vi "Credit Update.vi"(8 "error in (no error)":errorcluster, 10 "Credit":dbl, 11 "UI Actor in":refnum<class "UI Actor.lvclass">) -> (0 "error out":errorcluster, 3 "UI Actor out":refnum<class "UI Actor.lvclass">)   [LabVIEW 2020, in "UI Actor.lvlib" / "UI Actor.lvclass"]
uses:
  UI Actor.lvclass
  UI Actor.lvclass/UI Actor.ctl
  Msg Messages/Update MSG Msg/Update MSG Msg.lvclass/Update MSG Msg.ctl
  <vilib>/ActorFramework/Message Enqueuer/Message Enqueuer.lvclass/Message Enqueuer.ctl
  <vilib>/ActorFramework/Message Enqueuer/Enqueue.vi
  Msg Messages/Update MSG Msg/Update MSG Msg.lvclass
  C:/Program Files/National Instruments/LabVIEW 2020/vi.lib/ActorFramework/Message/Message.lvclass
  <vilib>/ActorFramework/Message Priority Queue/Priority Enqueue.vi
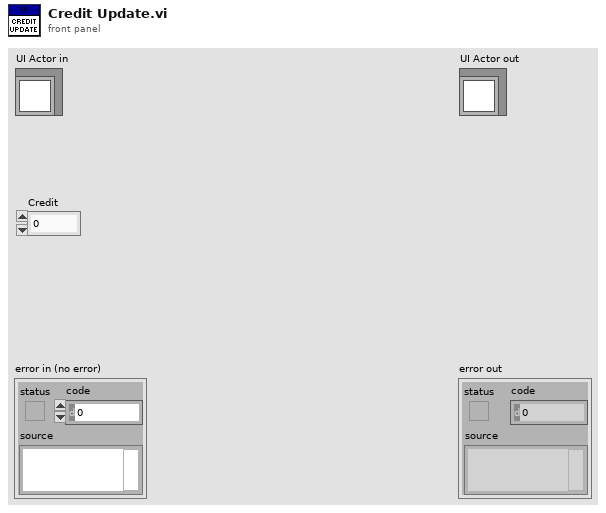
[diagram p1: front panel]
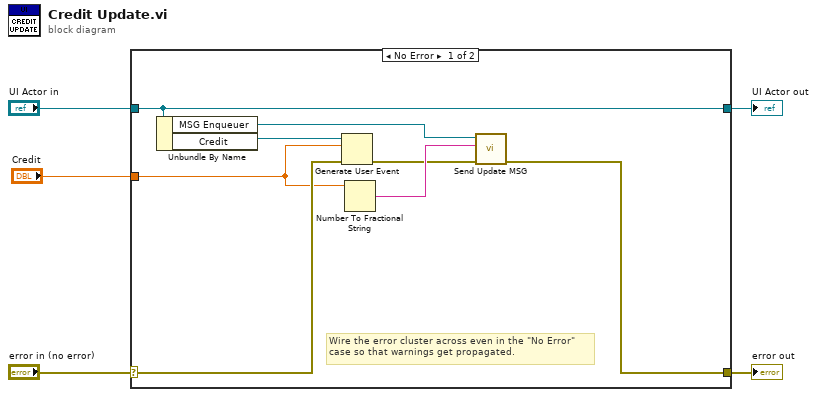
[diagram p0: block diagram]
diagram:
  n1 = case shown="No Error" "error in (no error)" {
    selector: "error in (no error)" -> [w13 w15]
    tunnel: [w6 w15] -> w4
    tunnel: [w12 w14] -> w2
    tunnel: "UI Actor in" -> [w12 w14]
    tunnel: "Credit" -> [w9 _]
    frame No Error {
      # "Wire the error cluster across even in the \"No Error\"\ncase so that warnings get propagated."
      n2 = Unbundle By Name(w12) -> ("MSG Enqueuer"=w10:refnum<class "Message Enqueuer.lvclass">, "Credit"=w11:refnum<user-event>)
      n3 = Generate User Event(user event=w11, event data cluster=w9, error in=w13) -> (error out=w7:errorcluster)  [unwired: 1 in, 1 out]
      n4 = Number To Fractional String(number=w9) -> (F-format string=w8:string)  [unwired: 3 in]
      n5 = call "Send Update MSG.vi"("error in (no error)"=w7, "Update MSG"=w8, "Message Enqueuer"=w10) -> ("error out"=w6:errorcluster)  [unwired: 7 in, 1 out]
    }
    frame Error {
    }
  }
  "error out" <- w4
  "UI Actor out" <- w2
